vi "Send Configure Msg.vi"(8 "error in":errorcluster, 10 "analog generation":T1={"output settings"={"channel list"="", "output rate"=0.0, "range"=0.0, "terminal configuration"=10106, "output impedance"=0.0, "common mode offset"=0.0, "pure tone mode"=FALSE}, "signal settings"={"signal type"=enum."Sine", "properties"=""}} {"output settings"."terminal configuration" items=["Default"=-1, "RSE"=10083, "Differential"=10106, "Pseudodifferential"=12529]}, 11 "Qbus in":refnum<class "Qbus.lvclass">) -> (0 "error out":errorcluster, 3 "Qbus out":refnum<class "Qbus.lvclass">)   [LabVIEW 2021, in "AnalogGeneration.lvlib"]
uses:
  AnalogGeneration.lvlib
  <vilib>/addons/Qbus/Qbus.lvclass
  controls/analog output settings.ctl
  controls/AudioGenTypeDefs.lvlib
  controls/signal type.ctl
  controls/signal settings.ctl
  controls/analog generation settings.ctl
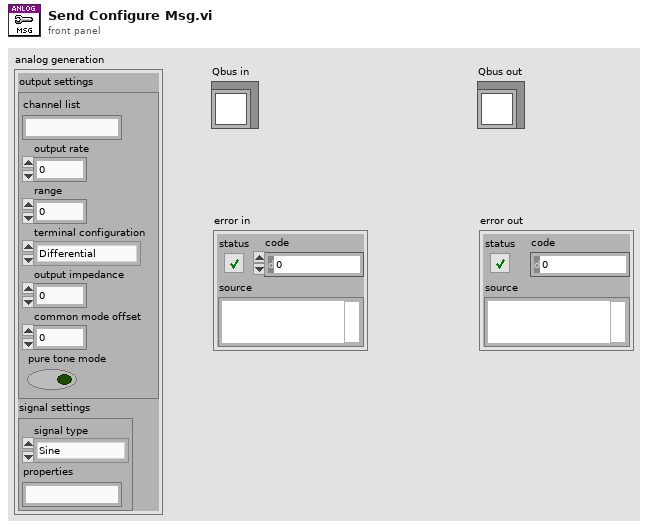
[diagram p1: front panel]
types:
  T1 = typedef "AudioGenTypeDefs.lvlib/analog generation settings.ctl" = cluster{"output settings":T2, "signal settings":T3}
  T2 = typedef "AudioGenTypeDefs.lvlib/analog output settings.ctl" = cluster{"channel list":string, "output rate":dbl, "range":dbl, "terminal configuration":i32, "output impedance":dbl, "common mode offset":dbl, "pure tone mode":bool}
  T3 = typedef "AudioGenTypeDefs.lvlib/signal settings.ctl" = cluster{"signal type":T4, "properties":string}
  T4 = typedef "AudioGenTypeDefs.lvlib/signal type.ctl" = enum16{"Sine", "Square", "Triangle", "White Noise", "Pink Noise", "Periodic Random Noise"}
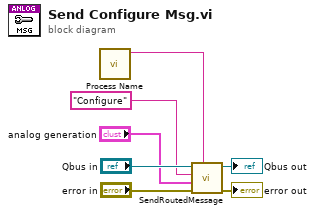
[diagram p0: block diagram]
diagram:
  n1 = call "Process Name.vi"() -> ("process name"=w2:string)  [unwired: 11 in]
  n2 = call <vilib>:"SendRoutedMessage.vi"("listener process"=w2, "error in (no error)"="error in", "message value"="analog generation", "message name"="Configure", "Qbus in"="Qbus in") -> ("error in (no error)"=→"error out":errorcluster, "Qbus out"=→"Qbus out":refnum<class "Qbus.lvclass">)  [unwired: 5 in]
